vi "Has Callbacks.vi"(8 "error in (no error)":errorcluster, 11 "Endpoint in":refnum<class "Endpoint.lvclass">) -> (0 "error out":errorcluster, 2 "Has Callbacks":bool, 3 "Endpoint out":refnum<class "Endpoint.lvclass">)   [LabVIEW 2020, in "Stream.lvlib" / "Endpoint.lvclass"]
uses:
  Endpoint.lvclass
  Endpoint.lvclass/Endpoint.ctl
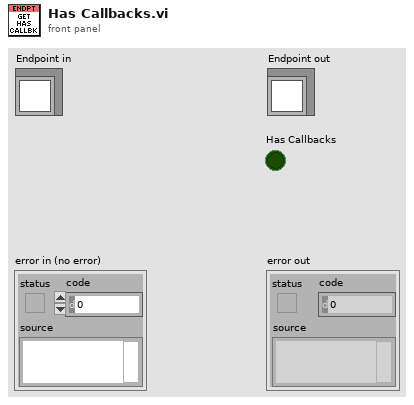
[diagram p1: front panel]
types:
  T1 = typedef "Stream.lvlib/Endpoint.lvclass/Ref Data.ctl" = cluster{"URI":refnum<class "URI.lvclass">, "State Callbacks":T2[], "Open":bool, "Mode":T3}
  T2 = typedef "Stream.lvlib/Endpoint.lvclass/State Callback.ctl" = cluster{"Owner":refnum<class>, "VI":refnum<vi>}
  T3 = typedef "Stream.lvlib/Mode.ctl" = enum16{"Raw", "Buffered", "LineTerm"}
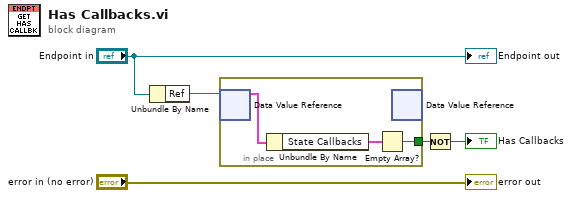
[diagram p0: block diagram]
diagram:
  n1 = Unbundle By Name("Endpoint in") -> ("Ref"=w4:refnum<data-value>)
  n2 = in-place {
    in-place-border: [w6] -> w2
    n3 = in-place-dvr #1(w4) -> (w8:T1)  [unwired: 1 out]
    n4 = Unbundle By Name(w8) -> ("State Callbacks"=w7:T2[])
    n5 = Empty Array?(array=w7) -> (empty?=w6:bool)
    n6 = in-place-dvr #1() -> ()  [unwired: 1 in, 2 out]
  }
  n7 = Not(x=w2) -> (.not. x?=→"Has Callbacks":bool)
  "error out" <- "error in (no error)"
  "Endpoint out" <- "Endpoint in"
